vi "TestFile.vi"(10 "status":bool, 11 "cancelled":bool) -> (3 "IsOpen":bool)   [LabVIEW 2018]
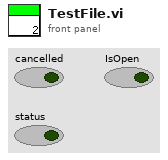
[diagram p1: front panel]
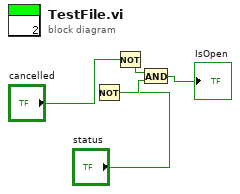
[diagram p0: block diagram]
diagram:
  n1 = Not(x="status") -> (.not. x?=w5:bool)
  n2 = Not(x="cancelled") -> (.not. x?=w3:bool)
  n3 = And(x=w3, y=w5) -> (x .and. y?=→"IsOpen":bool)
